vi "crio_FPGA_Plant_Dual_Motor.vi"() -> ()   [LabVIEW 2019]
uses:
  <vilib>/eio/EIOMethodNode/EIOMethodNode.xnode
  <vilib>/rvi/eio/common/nirviEmuTemplateMethod_errors.vi
  <vilib>/eio/EIONode/EIONode.xnode
  <vilib>/rvi/Analysis/control/PID/Typedef/niFpgaPID_OutputRange.ctl
  <vilib>/rvi/Analysis/control/PID/SubVIs/niFpgaPID_PIWrapper.vi
  <vilib>/rvi/Analysis/control/PID/Typedef/niFpgaPID_ManualControl.ctl
  <vilib>/rvi/Analysis/control/PID/Typedef/niFpgaPID_PIGains.ctl
panel:
  out "Loop Timer DAQ 3":u32=1 caption="Loop Time(uSec)"
  in  "stop":bool
  in  "Debug: ConnectorA/DIO15 Load":bool
  in  "Debug: ConnectorA/DIO14 Load":bool
  in  "Encoder Debug Load":bool
  in  "Position Reset Load":bool
  out "Position (Counts) Load":i64
  out "Load B":bool
  out "Load A":bool
  out "Load B'":bool
  out "Load A'":bool
  out "Acceleration (Counts/Interval) Load":i32
  out "Velocity (Counts/Interval) Load":i32
  out "ControllerPWM Output Load":sgl
  in  "manual control Load":T1 {"manual input (0)" scale=-1.0..1.0}
  in  "setpoint Load":i32
  in  "gains load":T2 {"proportional gain" step=0.125}
  out "ControllerPWM Output":sgl
  in  "manual control":T1 {"manual input (0)" scale=-1.0..1.0}
  in  "setpoint":i32
  in  "gains":T2 {"proportional gain" step=0.125}
  in  "Debug: ConnectorA/DIO15":bool
  in  "Debug: ConnectorA/DIO14":bool
  in  "Encoder Debug":bool
  in  "Loop Timer DAQ":u32=1 caption="Loop Time(uSec)"
  in  "Position Reset":bool
  out "Position (Counts)":i64
  out "B":bool
  out "A":bool
  out "B'":bool
  out "A'":bool
  in  "Velocity Interval (uSec)":u32=1000
  out "Acceleration (Counts/Interval)":i32
  out "Velocity (Counts/Interval)":i32
  in  "DC PWM Period (microsec)":i16=50
  # "DRV8256 Specs:\n\n0 0: Brake Low\n1 1: Brake High\nPWM 0\n0 PWM"
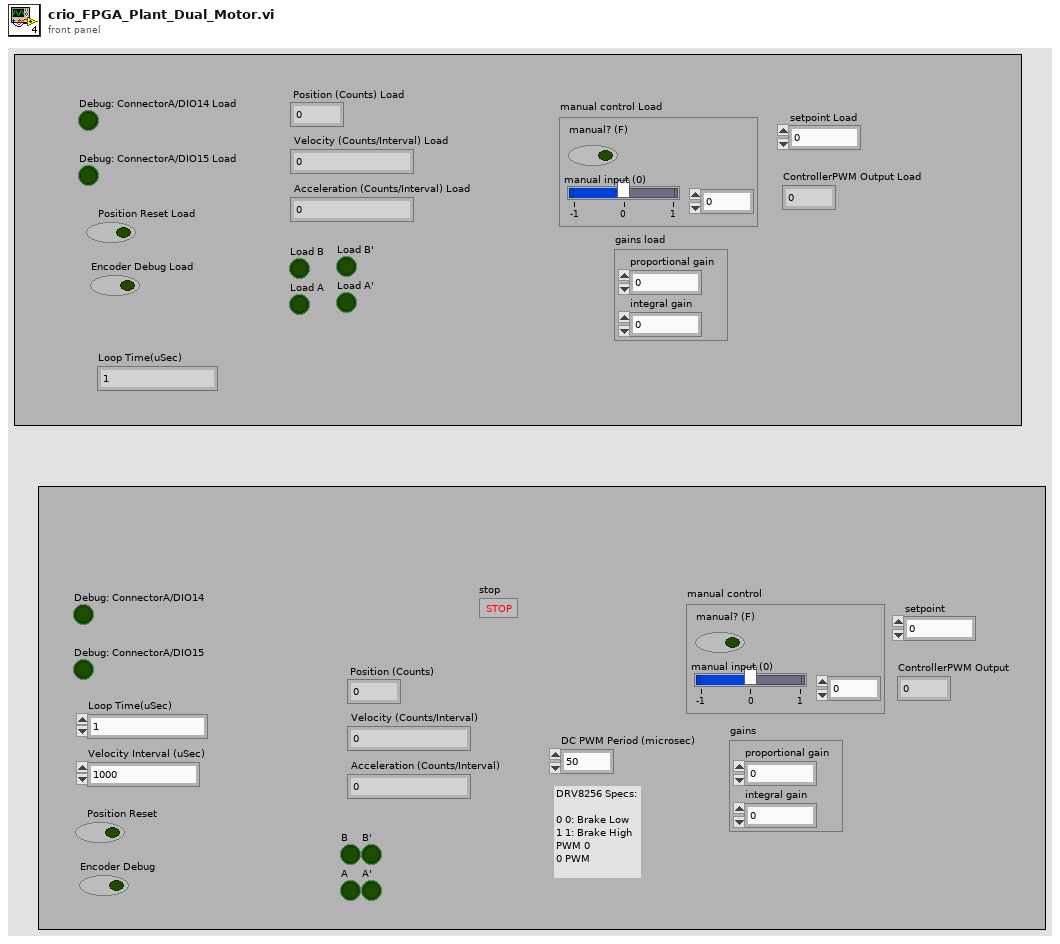
[diagram p1: front panel]
types:
  T1 = typedef "niFpgaPID_ManualControl.ctl" = cluster{"manual? (F)":bool, "manual input (0)":sgl}
  T2 = typedef "niFpgaPID_PIGains.ctl" = cluster{"proportional gain":sgl, "integral gain":sgl}
  T3 = typedef "niFpgaPID_OutputRange.ctl" = cluster{"output high (Inf)":sgl, "output low (-Inf)":sgl}
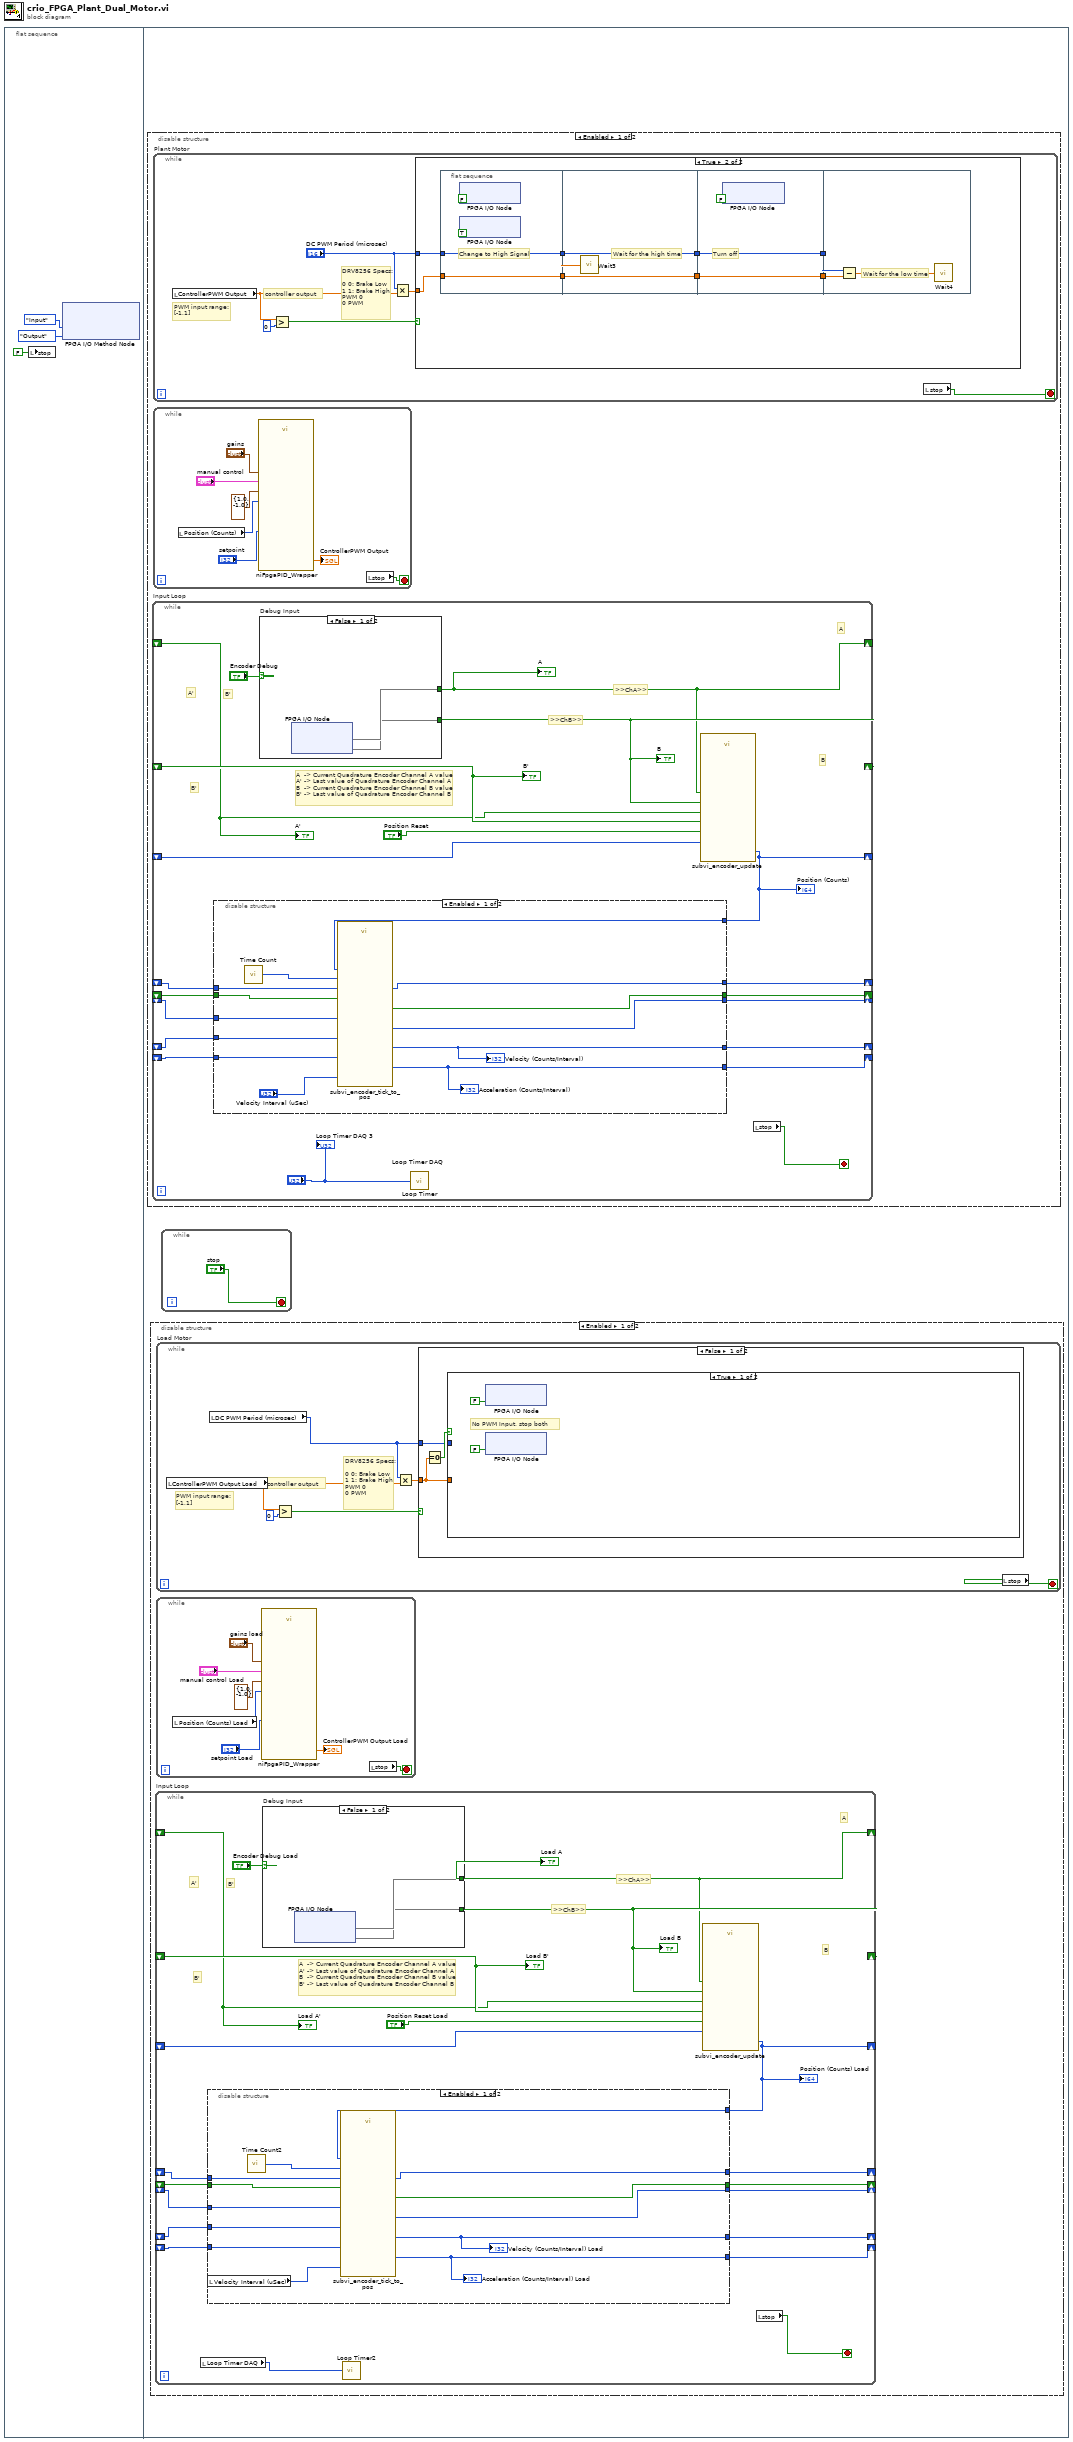
[diagram p0: block diagram]
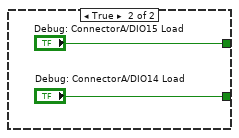
[diagram p3: hidden frame]
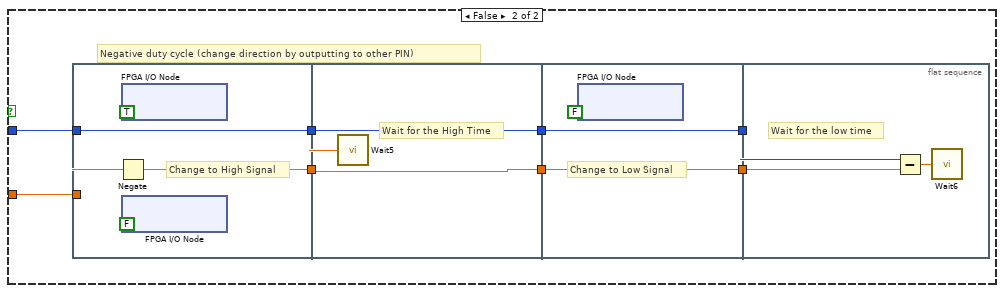
[diagram p4: hidden frame]
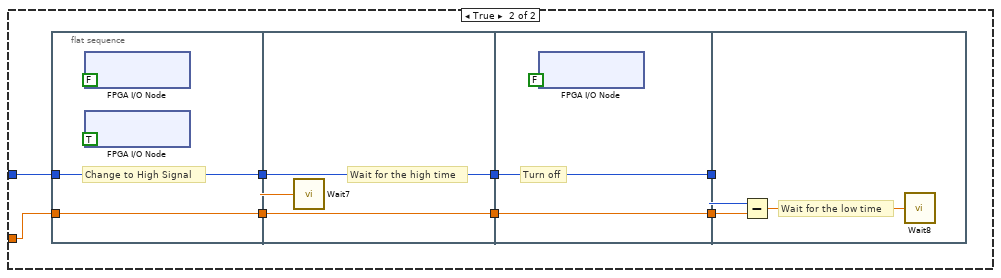
[diagram p5: hidden frame]
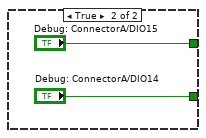
[diagram p8: hidden frame]
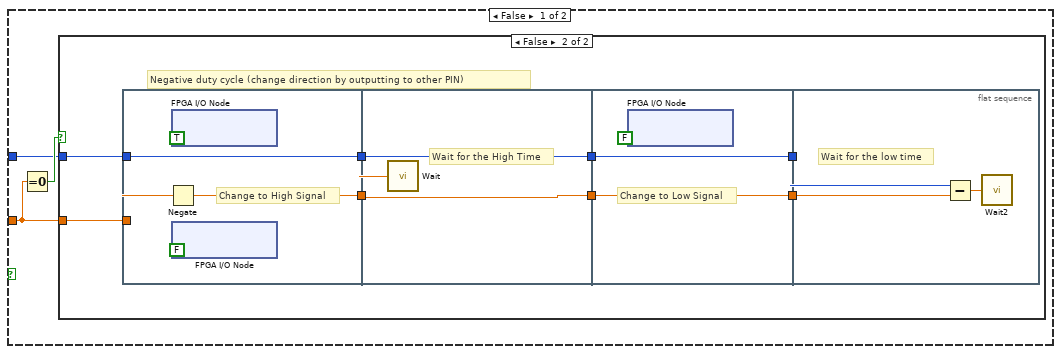
[diagram p9: hidden frame]
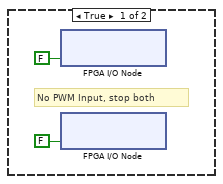
[diagram p10: hidden frame]
diagram:
  n1 = flat-sequence {
    frame #0 {
      n2 = local write "stop"(FALSE ("stop")) -> ()
      n3 = xnode "FPGA I/O Method Node"("DIO 7:4"=enum8{"No Change", "Input", "Output"}."Input", "DIO 3:0"=enum8{"No Change", "Input", "Output"}."Output") -> ()  [unwired: 1 in, 1 out]
    }
    frame #1 {
      n4 = disable-structure shown="Enabled" {
        frame Enabled {
          n5 = while "Input Loop" {
            shift-right: [w121] -> _
            shift-left: _ -> [w124]
            shift-right: [w120] -> _
            shift-left: _ -> [w123]
            shift-right: [w116] -> _
            shift-left: _ -> [w122]
            shift-right: [w109] -> _
            shift-left: _ -> [w119]
            shift-right: [w110] -> _
            shift-left: _ -> [w118]
            shift-right: [w117] -> _
            shift-left: _ -> [w115]
            shift-right: [w114] -> _
            shift-left: _ -> [w113]
            shift-right: [w112] -> _
            shift-left: _ -> [w111]
            stop <- w108 stop-if-true
            # "B'"
            # ">>ChB>>"
            # ">>ChA>>"
            # "A'"
            # "A  -> Current Quadrature Encoder Channel A value\nA' -> Last value of Quadrature Encoder Channel A\nB  -> Current Quadrature Encoder Channel B value\nB' -> Last value of Quadrature Encoder Channel B"
            # "B'"
            # "B"
            # "A"
            n6 = case "Debug Input" shown="False" "Encoder Debug" {
              tunnel: [w142 "Debug: ConnectorA/DIO15"] -> w120
              tunnel: [w141 "Debug: ConnectorA/DIO14"] -> w121
              frame False {
                n7 = xnode "FPGA I/O Node"() -> ("Mod7/DIO4"=w142, "Mod7/DIO5"=w141)  [unwired: 2 in, 2 out]
              }
              frame True {
              }
            }
            "B" <- w121
            "A" <- w120
            n8 = call "Loop Timer"("Count(uSec)"="Loop Timer DAQ") -> ()  [unwired: 1 out]
            n9 = call "subvi_encoder_update.vi"("Position Reset"="Position Reset", "Tick'"=w122, "A"=w120, "B'"=w124, "A'"=w123, "B"=w121) -> ("Tick"=w116:i32)  [unwired: 5 in]
            "Position (Counts)" <- w116
            n10 = disable-structure shown="Enabled" {
              disable-tunnel: w119 -> [w139 _]
              disable-tunnel: w118 -> [w138 _]
              disable-tunnel: [w137 _] -> w117
              disable-tunnel: w116 -> [w136 _]
              disable-tunnel: w115 -> [w135 _]
              disable-tunnel: [w134 _] -> w114
              disable-tunnel: w113 -> [w133 _]
              disable-tunnel: [w132 _] -> w112
              disable-tunnel: w111 -> [w131 _]
              disable-tunnel: [w129 _] -> w110
              disable-tunnel: [w128 _] -> w109
              frame Enabled {
                n11 = call "Time Count"() -> ("Tick Count(uSec)"=w130:u32)
                n12 = call "subvi_encoder_tick_to_pos.vi"("Velocity Interval (uSec)"="Velocity Interval (uSec)", "Raw Tick"=w136, "Waited?'"=w133, "Tick Count(uSec)'"=w131, "p'"=w135, "Time Count"=w130, "a'"=w138, "v'"=w139) -> ("Waited?"=w134:bool, "Tick Count(uSec)"=w132:u32, "p"=w137:i32, "a"=w129:i32, "v"=w128:i32)  [unwired: 3 in]
                "Acceleration (Counts/Interval)" <- w129
                "Velocity (Counts/Interval)" <- w128
              }
              frame Disabled {
              }
            }
            n13 = local read "stop"() -> (w108:bool)
            "B'" <- w124
            "A'" <- w123
            "Loop Timer DAQ 3" <- "Loop Timer DAQ"
          }
          n14 = while "Plant Motor" {
            stop <- w145 stop-if-true
            # "PWM input range:\n[-1,1]"
            # "DRV8256 Specs:\n\n0 0: Brake Low\n1 1: Brake High\nPWM 0\n0 PWM"
            # "controller output"
            n15 = local read "ControllerPWM Output"() -> (w146:sgl)
            n16 = Greater?(x=w146, y=i16 0) -> (0:w149:bool)
            n17 = Multiply(x="DC PWM Period (microsec)", y=w146) -> (x*y=w148:sgl)
            n18 = case shown="True" w149 {
              tunnel: w148 -> [w153 w184]
              tunnel: "DC PWM Period (microsec)" -> [w151 w183]
              frame False {
                n19 = Equal To 0?(x=w153) -> (x = 0?=w152:bool)
                n20 = case shown="False" w152 {
                  tunnel: w153 -> [_ w163]
                  tunnel: w151 -> [_ w156]
                  frame True {
                    # "No PWM Input, stop both"
                    n21 = xnode "FPGA I/O Node"("Mod7/DIO1"=FALSE) -> ()  [unwired: 1 in, 1 out]
                    n22 = xnode "FPGA I/O Node"("Mod7/DIO0"=FALSE) -> ()  [unwired: 1 in, 1 out]
                  }
                  frame False {
                    # "Negative duty cycle (change direction by outputting to other PIN)"
                    n23 = flat-sequence {
                      tunnel: w163 -> [w166]
                      tunnel: [w165] -> w162
                      tunnel: [w164] -> w157
                      tunnel: w156 -> [w164]
                      tunnel: w162 -> [w170]
                      tunnel: [w170] -> w161
                      tunnel: [w169] -> w158
                      tunnel: w157 -> [w169]
                      tunnel: w161 -> [w172]
                      tunnel: [w172] -> w160
                      tunnel: [w171] -> w159
                      tunnel: w158 -> [w171]
                      tunnel: w160 -> [w176]
                      tunnel: w159 -> [w175]
                      frame #0 {
                        # "Change to High Signal"
                        n24 = Negate(x=w166) -> (-x=w165:sgl)
                        n25 = xnode "FPGA I/O Node"("Mod7/DIO1"=TRUE) -> ()  [unwired: 1 in, 1 out]
                        n26 = xnode "FPGA I/O Node"("Mod7/DIO0"=FALSE) -> ()  [unwired: 1 in, 1 out]
                      }
                      frame #1 {
                        # "Wait for the High Time"
                        n27 = call "Wait"("Count(uSec)"=w170) -> ()  [unwired: 1 out]
                      }
                      frame #2 {
                        # "Change to Low Signal"
                        n28 = xnode "FPGA I/O Node"("Mod7/DIO1"=FALSE) -> ()  [unwired: 1 in, 1 out]
                      }
                      frame #3 {
                        # "Wait for the low time"
                        n29 = Subtract(x=w175, y=w176) -> (x-y=w174:sgl)
                        n30 = call "Wait2"("Count(uSec)"=w174) -> ()  [unwired: 1 out]
                      }
                    }
                  }
                }
              }
              frame True {
                n31 = flat-sequence {
                  tunnel: w184 -> [w185]
                  tunnel: w183 -> [w186]
                  tunnel: [w186] -> w180
                  tunnel: [w185] -> w179
                  tunnel: [w190] -> w181
                  tunnel: w180 -> [w190]
                  tunnel: w179 -> [w189]
                  tunnel: [w189] -> w178
                  tunnel: [w192] -> w182
                  tunnel: w181 -> [w192]
                  tunnel: w178 -> [w191]
                  tunnel: [w191] -> w177
                  tunnel: w182 -> [w196]
                  tunnel: w177 -> [w194]
                  frame #0 {
                    # "Change to High Signal"
                    n32 = xnode "FPGA I/O Node"("Mod7/DIO1"=FALSE ("ConnectorB/DIO9")) -> ()  [unwired: 1 in, 1 out]
                    n33 = xnode "FPGA I/O Node"("Mod7/DIO0"=TRUE) -> ()  [unwired: 1 in, 1 out]
                  }
                  frame #1 {
                    # "Wait for the high time"
                    n34 = call "Wait3"("Count(uSec)"=w189) -> ()  [unwired: 1 out]
                  }
                  frame #2 {
                    # "Turn off"
                    n35 = xnode "FPGA I/O Node"("Mod7/DIO0"=FALSE) -> ()  [unwired: 1 in, 1 out]
                  }
                  frame #3 {
                    # "Wait for the low time"
                    n36 = Subtract(x=w196, y=w194) -> (x-y=w195:sgl)
                    n37 = call "Wait4"("Count(uSec)"=w195) -> ()  [unwired: 1 out]
                  }
                }
              }
            }
            n38 = local read "stop"() -> (w145:bool)
          }
          n39 = while {
            stop <- w107 stop-if-true
            n40 = local read "Position (Counts)"() -> (w106:i64)
            n41 = call-poly <vilib>:"niFpgaPID_Wrapper.vi"("setpoint"="setpoint", "process variable"=w106, "manual control"="manual control", "gains"="gains", "output range"=T3 {"output high (Inf)"=1.0, "output low (-Inf)"=-1.0}) -> ("output"=→"ControllerPWM Output":sgl)  [unwired: 8 in, 2 out]
            n42 = local read "stop"() -> (w107:bool)
          }
        }
        frame Disabled {
        }
      }
      n43 = disable-structure shown="Enabled" {
        frame Enabled {
          n44 = while "Input Loop" {
            shift-right: [w26] -> _
            shift-left: _ -> [w29]
            shift-right: [w25] -> _
            shift-left: _ -> [w28]
            shift-right: [w21] -> _
            shift-left: _ -> [w27]
            shift-right: [w14] -> _
            shift-left: _ -> [w24]
            shift-right: [w15] -> _
            shift-left: _ -> [w23]
            shift-right: [w22] -> _
            shift-left: _ -> [w20]
            shift-right: [w19] -> _
            shift-left: _ -> [w18]
            shift-right: [w17] -> _
            shift-left: _ -> [w16]
            stop <- w12 stop-if-true
            # "B'"
            # ">>ChB>>"
            # ">>ChA>>"
            # "A'"
            # "A  -> Current Quadrature Encoder Channel A value\nA' -> Last value of Quadrature Encoder Channel A\nB  -> Current Quadrature Encoder Channel B value\nB' -> Last value of Quadrature Encoder Channel B"
            # "B'"
            # "B"
            # "A"
            n45 = local read "Loop Timer DAQ"() -> (w13:u32)
            n46 = case "Debug Input" shown="False" "Encoder Debug Load" {
              tunnel: [w46 "Debug: ConnectorA/DIO15 Load"] -> w25
              tunnel: [w45 "Debug: ConnectorA/DIO14 Load"] -> w26
              frame False {
                n47 = xnode "FPGA I/O Node"() -> ("Mod7/DIO6"=w46, "Mod7/DIO7"=w45)  [unwired: 2 in, 2 out]
              }
              frame True {
              }
            }
            "Load B" <- w26
            "Load A" <- w25
            n48 = call "Loop Timer2"("Count(uSec)"=w13) -> ()  [unwired: 1 out]
            n49 = call "subvi_encoder_update.vi"("Position Reset"="Position Reset Load", "Tick'"=w27, "A"=w25, "B'"=w29, "A'"=w28, "B"=w26) -> ("Tick"=w21:i32)  [unwired: 5 in]
            "Position (Counts) Load" <- w21
            n50 = disable-structure shown="Enabled" {
              disable-tunnel: w24 -> [w44 _]
              disable-tunnel: w23 -> [w43 _]
              disable-tunnel: [w42 _] -> w22
              disable-tunnel: w21 -> [w41 _]
              disable-tunnel: w20 -> [w40 _]
              disable-tunnel: [w39 _] -> w19
              disable-tunnel: w18 -> [w38 _]
              disable-tunnel: [w37 _] -> w17
              disable-tunnel: w16 -> [w36 _]
              disable-tunnel: [w34 _] -> w15
              disable-tunnel: [w33 _] -> w14
              frame Enabled {
                n51 = local read "Velocity Interval (uSec)"() -> (w32:u32)
                n52 = call "Time Count2"() -> ("Tick Count(uSec)"=w35:u32)
                n53 = call "subvi_encoder_tick_to_pos.vi"("Velocity Interval (uSec)"=w32, "Raw Tick"=w41, "Waited?'"=w38, "Tick Count(uSec)'"=w36, "p'"=w40, "Time Count"=w35, "a'"=w43, "v'"=w44) -> ("Waited?"=w39:bool, "Tick Count(uSec)"=w37:u32, "p"=w42:i32, "a"=w34:i32, "v"=w33:i32)  [unwired: 3 in]
                "Acceleration (Counts/Interval) Load" <- w34
                "Velocity (Counts/Interval) Load" <- w33
              }
              frame Disabled {
              }
            }
            n54 = local read "stop"() -> (w12:bool)
            "Load B'" <- w29
            "Load A'" <- w28
          }
          n55 = while "Load Motor" {
            stop <- w49 stop-if-true
            # "PWM input range:\n[-1,1]"
            # "DRV8256 Specs:\n\n0 0: Brake Low\n1 1: Brake High\nPWM 0\n0 PWM"
            # "controller output"
            n56 = local read "ControllerPWM Output Load"() -> (w51:sgl)
            n57 = local read "DC PWM Period (microsec)"() -> (w50:i16)
            n58 = Greater?(x=w51, y=i16 0) -> (0:w53:bool)
            n59 = Multiply(x=w50, y=w51) -> (x*y=w52:sgl)
            n60 = case shown="False" w53 {
              tunnel: w52 -> [w57 w88]
              tunnel: w50 -> [w55 w87]
              frame False {
                n61 = Equal To 0?(x=w57) -> (x = 0?=w56:bool)
                n62 = case shown="True" w56 {
                  tunnel: w57 -> [_ w67]
                  tunnel: w55 -> [_ w60]
                  frame True {
                    # "No PWM Input, stop both"
                    n63 = xnode "FPGA I/O Node"("Mod7/DIO2"=FALSE) -> ()  [unwired: 1 in, 1 out]
                    n64 = xnode "FPGA I/O Node"("Mod7/DIO3"=FALSE) -> ()  [unwired: 1 in, 1 out]
                  }
                  frame False {
                    # "Negative duty cycle (change direction by outputting to other PIN)"
                    n65 = flat-sequence {
                      tunnel: w67 -> [w70]
                      tunnel: [w69] -> w66
                      tunnel: [w68] -> w61
                      tunnel: w60 -> [w68]
                      tunnel: w66 -> [w74]
                      tunnel: [w74] -> w65
                      tunnel: [w73] -> w62
                      tunnel: w61 -> [w73]
                      tunnel: w65 -> [w76]
                      tunnel: [w76] -> w64
                      tunnel: [w75] -> w63
                      tunnel: w62 -> [w75]
                      tunnel: w64 -> [w80]
                      tunnel: w63 -> [w79]
                      frame #0 {
                        # "Change to High Signal"
                        n66 = Negate(x=w70) -> (-x=w69:sgl)
                        n67 = xnode "FPGA I/O Node"("Mod7/DIO3"=TRUE) -> ()  [unwired: 1 in, 1 out]
                        n68 = xnode "FPGA I/O Node"("Mod7/DIO2"=FALSE) -> ()  [unwired: 1 in, 1 out]
                      }
                      frame #1 {
                        # "Wait for the High Time"
                        n69 = call "Wait5"("Count(uSec)"=w74) -> ()  [unwired: 1 out]
                      }
                      frame #2 {
                        # "Change to Low Signal"
                        n70 = xnode "FPGA I/O Node"("Mod7/DIO3"=FALSE) -> ()  [unwired: 1 in, 1 out]
                      }
                      frame #3 {
                        # "Wait for the low time"
                        n71 = Subtract(x=w79, y=w80) -> (x-y=w78:sgl)
                        n72 = call "Wait6"("Count(uSec)"=w78) -> ()  [unwired: 1 out]
                      }
                    }
                  }
                }
              }
              frame True {
                n73 = flat-sequence {
                  tunnel: w88 -> [w89]
                  tunnel: w87 -> [w90]
                  tunnel: [w90] -> w84
                  tunnel: [w89] -> w83
                  tunnel: [w94] -> w85
                  tunnel: w84 -> [w94]
                  tunnel: w83 -> [w93]
                  tunnel: [w93] -> w82
                  tunnel: [w96] -> w86
                  tunnel: w85 -> [w96]
                  tunnel: w82 -> [w95]
                  tunnel: [w95] -> w81
                  tunnel: w86 -> [w100]
                  tunnel: w81 -> [w98]
                  frame #0 {
                    # "Change to High Signal"
                    n74 = xnode "FPGA I/O Node"("Mod7/DIO3"=FALSE ("ConnectorB/DIO9")) -> ()  [unwired: 1 in, 1 out]
                    n75 = xnode "FPGA I/O Node"("Mod7/DIO2"=TRUE) -> ()  [unwired: 1 in, 1 out]
                  }
                  frame #1 {
                    # "Wait for the high time"
                    n76 = call "Wait7"("Count(uSec)"=w93) -> ()  [unwired: 1 out]
                  }
                  frame #2 {
                    # "Turn off"
                    n77 = xnode "FPGA I/O Node"("Mod7/DIO2"=FALSE) -> ()  [unwired: 1 in, 1 out]
                  }
                  frame #3 {
                    # "Wait for the low time"
                    n78 = Subtract(x=w100, y=w98) -> (x-y=w99:sgl)
                    n79 = call "Wait8"("Count(uSec)"=w99) -> ()  [unwired: 1 out]
                  }
                }
              }
            }
            n80 = local read "stop"() -> (w49:bool)
          }
          n81 = while {
            stop <- w5 stop-if-true
            n82 = local read "Position (Counts) Load"() -> (w11:i64)
            n83 = call-poly <vilib>:"niFpgaPID_Wrapper.vi"("setpoint"="setpoint Load", "process variable"=w11, "manual control"="manual control Load", "gains"="gains load", "output range"=T3 {"output high (Inf)"=1.0, "output low (-Inf)"=-1.0}) -> ("output"=→"ControllerPWM Output Load":sgl)  [unwired: 8 in, 2 out]
            n84 = local read "stop"() -> (w5:bool)
          }
        }
        frame Disabled {
        }
      }
      n85 = while {
        stop <- "stop" stop-if-true
      }
    }
  }
